vi "ARCHIVE ITEM.vi"(10 "REFERENCES":T2, 11 "ITEM DATA IN":T1) -> ()   [LabVIEW 2019]
uses:
  Controls/References Cluster.ctl
  <vilib>/userDefined/High Color/IMAQdx.ctl
  Controls/Custom Calendar/Custom Calendar.xctl
  Controls/Table Data Types/Inventory Archive Data Type.ctl
  Controls/Table Data Types/Checked In Archive Data Type.ctl
  <vilib>/addons/database/Connection.llb/DB Tools Open Connec (String).vi
  <vilib>/addons/database/NI_Database_API.lvlib
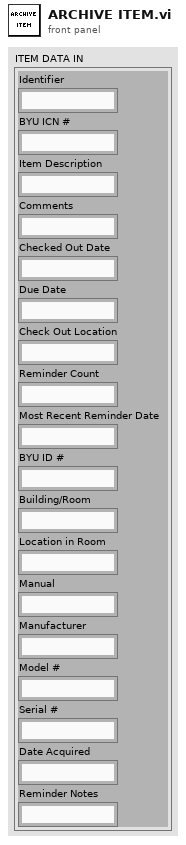
[diagram p1: front panel]
types:
  T1 = cluster{"Identifier":string, "BYU ICN #":string, "Item Description":string, "Comments":string, "Checked Out Date":string, "Due Date":string, "Check Out Location":string, "Reminder Count":string, "Most Recent Reminder Date":string, "BYU ID #":string, "Building/Room":string, "Location in Room":string, "Manual":string, "Manufacturer":string, "Model #":string, "Serial #":string, "Date Acquired":string, "Reminder Notes":string}
  T2 = typedef "References Cluster.ctl" = cluster{"MAIN PAGES":refnum<vi>, "ADD/EDIT ITEM REFERENCES":cluster{"Identifier":refnum<vi>, "BYU ICN #":refnum<vi>, "Item Description":refnum<vi>, "Comments":refnum<vi>, "Checked Out Date":refnum<vi>, "Due Date":refnum<vi>, "Check Out Location":refnum<vi>, "Reminder Count":refnum<vi>, "Most Recent Reminder Date":refnum<vi>, "BYU ID #":refnum<vi>, "Building/Room":refnum<vi>, "Location in Room":refnum<vi>, "Manual":refnum<vi>, "Manufacturer":refnum<vi>, "Model #":refnum<vi>, "Serial #":refnum<vi>, "Date Acquired":refnum<vi>, "ADD/EDIT ITEM LABEL":refnum<vi>, "ARCHIVE ITEM":refnum<vi>, "Archive Item Inputs":refnum<vi>, "Reminder Notes":refnum<vi>}, "ADD/EDIT USER REFERENCES":cluster{"BYU ID # (##-###-####)":refnum<vi>, "First Name":refnum<vi>, "Last Name":refnum<vi>, "Phone Number (###-###-####)":refnum<vi>, "Email":refnum<vi>, "Department":refnum<vi>, "Graduation Status":refnum<vi>, "Anticipated Graduation Year":refnum<vi>, "Credit Score":refnum<vi>, "Date Added":refnum<vi>, "Graduation Clearance Date":refnum<vi>, "Picture File Name":refnum<vi>, "ADD/EDIT USER LABEL":refnum<vi>, "Department Map":refnum<vi>, "Status Map":refnum<vi>, "Anticipated Graduation Year Map":refnum<vi>, "User Agreement":refnum<vi>, "User Comments":refnum<vi>, "Camera":refnum<vi>}, "RETURN ITEM REFERENCES":cluster{"Item or Person:":refnum<vi>, "Search Return Results":refnum<vi>, "What are you searching for?":refnum<vi>}, "SEARCH DATABASE REFERENCES":cluster{"What to Search For:":refnum<vi>, "Where to Search":refnum<vi>, "Column to Search In":refnum<vi>, "Column to Sort By":refnum<vi>, "Search Database Results":refnum<vi>, "Inventory Column Selector":refnum<vi>, "User Column Selector":refnum<vi>, "Inventory Archive Column Selector":refnum<vi>, "User Archive Column Selector":refnum<vi>, "Sales Tracking Column Selector":refnum<vi>, "Checked In Archive Column Selector":refnum<vi>, "Restore User":refnum<vi>, "Date Range":refnum<vi>, "Dates Less Than":refnum<vi>, "Dates Greater Than":refnum<vi>, "Search Print Receipt":refnum<vi>, "Edit Sale Description":refnum<vi>}, "USER ITEMS REFERENCES":cluster{"USER'S INFORMATION":refnum<vi>, "User's Checked Out Items":refnum<vi>, "User Info Comments":refnum<vi>, "SEE USER INFO COMMENTS":refnum<vi>}, "EDIT ITEMS REFERENCES":cluster{"New Check Out Location":refnum<vi>, "Items to Edit":refnum<vi>, "Edit Items Due Date":refnum<vi>, "New Reminder Notes":refnum<vi>, "New Item Description":refnum<vi>}, "CHECK OUT ITEMS REFERENCES":cluster{"Enter Item:":refnum<vi>, "Check Out Items Due Date":refnum<vi>, "Check Out Location":refnum<vi>, "Items to be Checked Out":refnum<vi>, "Possible Items":refnum<vi>, "Altered Item Description":refnum<vi>}, "TRANSFER ITEMS REFERENCES":cluster{"Search Parameter":refnum<vi>, "What to Match":refnum<vi>, "Matching Individuals":refnum<vi>, "Items to be Transferred":refnum<vi>}, "SETTINGS REFERENCES":cluster{"PSC Database Settings":refnum<vi>, "PSC Sales Item Spreadsheet":refnum<vi>}, "PSC SALES REFERENCES":cluster{"BYU ID CARD #":refnum<vi>, "Sale Description":refnum<vi>, "Scan or Enter Item Name":refnum<vi>, "Items to be Sold":refnum<vi>, "Grand Total":refnum<vi>, "Item List":refnum<vi>}}
  T3 = typedef "Inventory Archive Data Type.ctl" = cluster{"Date Disposed":string, "Disposal Method":string, "Auction #":string, "Date Inventory Office Emailed":string, "Disposal Notes":string, "Identifier":string, "BYU ICN #":string, "Item Description":string, "Comments":string, "Building/Room":string, "Location in Room":string, "Manual":string, "Manufacturer":string, "Model #":string, "Serial #":string, "Date Acquired":string}
  T4 = cluster{"Identifier":refnum<vi>, "BYU ICN #":refnum<vi>, "Item Description":refnum<vi>, "Comments":refnum<vi>, "Checked Out Date":refnum<vi>, "Due Date":refnum<vi>, "Check Out Location":refnum<vi>, "Reminder Count":refnum<vi>, "Most Recent Reminder Date":refnum<vi>, "BYU ID #":refnum<vi>, "Building/Room":refnum<vi>, "Location in Room":refnum<vi>, "Manual":refnum<vi>, "Manufacturer":refnum<vi>, "Model #":refnum<vi>, "Serial #":refnum<vi>, "Date Acquired":refnum<vi>, "ADD/EDIT ITEM LABEL":refnum<vi>, "ARCHIVE ITEM":refnum<vi>, "Archive Item Inputs":refnum<vi>, "Reminder Notes":refnum<vi>}
  T5 = typedef "NI_Database_API.lvlib/Conn ObjectReference.ctl" = refnum<k1>
  T6 = typedef "Checked In Archive Data Type.ctl" = cluster{"Identifier":string, "BYU ICN #":string, "Item Description":string, "Comments":string, "Checked Out Date":string, "Due Date":string, "Check Out Location":string, "Reminder Count":i32, "Most Recent Reminder Date":string, "BYU ID #":string, "Building/Room":string, "Location in Room":string, "Manual":string, "Manufacturer":string, "Model #":string, "Serial #":string, "Date Acquired":string, "Date Returned":string, "Reminder Notes":string}
  T7 = cluster{"Disposal Date":string, "Disposal Method":u16, "Auction # / Other":string, "Date Disposal Email Sent":string, "Disposal Notes":string}
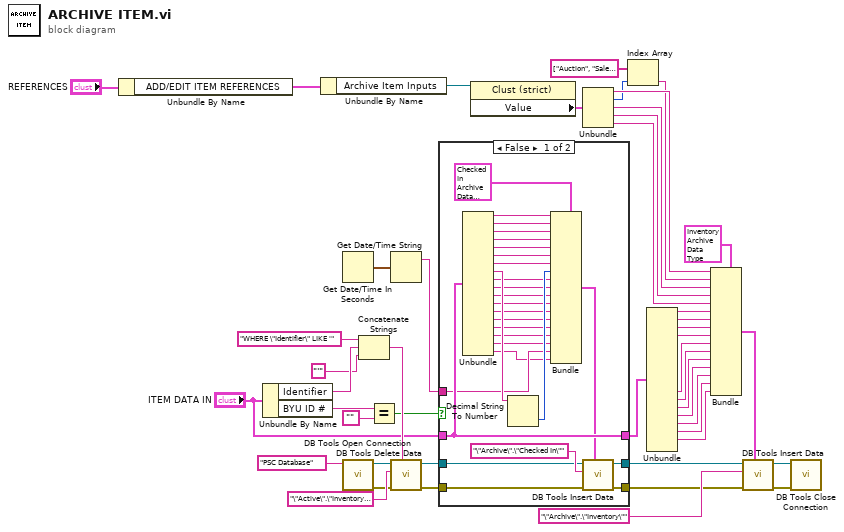
[diagram p0: block diagram]
diagram:
  n1 = Unbundle By Name("REFERENCES") -> ("ADD/EDIT ITEM REFERENCES"=w27:T4)
  n2 = Unbundle By Name("ITEM DATA IN") -> ("Identifier"=w44:string, "BYU ID #"=w39:string)
  n3 = Unbundle By Name(w27) -> ("Archive Item Inputs"=w26:refnum<vi>)
  n4 = Get Date/Time In Seconds() -> (seconds since 1Jan1904=w29:timestamp)
  n5 = call-poly <vilib>:"DB Tools Open Connection.vi"("connection information"="PSC Database") -> ("error out"=w41:errorcluster, "connection reference"=w40:T5)  [unwired: 7 in]
  n6 = Concatenate Strings("WHERE \"Identifier\" LIKE '" ("string"), w44, "'" ("string")) -> (w43:string)
  n7 = Equal?(x=w39, y="") -> (x = y?=w37:bool)
  n8 = Get Date/Time String(seconds (now)=w29) -> (date string=w28:string)  [unwired: 2 in, 1 out]
  n9 = call <vilib>:"DB Tools Delete Data.vi"("condition"=w43, "error in (no error)"=w41, "table"="\"Active\".\"Inventory\"" ("string"), "connection reference"=w40) -> ("error out"=w35:errorcluster, "connection reference out"=w36:T5)  [unwired: 6 in]
  n10 = case shown="False" w37 {
    tunnel: w36 -> [w73 w77]
    tunnel: w35 -> [w72 w76]
    tunnel: [w71 w77] -> w32
    tunnel: [w70 w76] -> w33
    tunnel: "ITEM DATA IN" -> [w69 w75]
    tunnel: [w69 w75] -> w24
    tunnel: w28 -> [w48 _]
    frame False {
      n11 = Unbundle(w69) -> ("Identifier"=w66:string, "BYU ICN #"=w65:string, "Item Description"=w64:string, "Comments"=w63:string, "Checked Out Date"=w62:string, "Due Date"=w61:string, "Check Out Location"=w60:string, "Reminder Count"=w59:string, "Most Recent Reminder Date"=w57:string, "BYU ID #"=w56:string, "Building/Room"=w55:string, "Location in Room"=w54:string, "Manual"=w53:string, "Manufacturer"=w52:string, "Model #"=w51:string, "Serial #"=w50:string, "Date Acquired"=w49:string, "Reminder Notes"=w47:string)
      n12 = Decimal String To Number(string=w59) -> (number=w58:i32)  [unwired: 2 in, 1 out]
      n13 = Bundle(cluster=T6 {"Identifier"="", "BYU ICN #"="", "Item Description"="", "Comments"="", "Checked Out Date"="", "Due Date"="", "Check Out Location"="", "Reminder Count"=0, "Most Recent Reminder Date"="", "BYU ID #"="", "Building/Room"="", "Location in Room"="", "Manual"="", "Manufacturer"="", "Model #"="", "Serial #"="", "Date Acquired"="", "Date Returned"="", "Reminder Notes"=""} ("CHECKED IN ARCHIVE DATA TYPE"), "Identifier"=w66, "BYU ICN #"=w65, "Item Description"=w64, "Comments"=w63, "Checked Out Date"=w62, "Due Date"=w61, "Check Out Location"=w60, "Reminder Count"=w58, "Most Recent Reminder Date"=w57, "BYU ID #"=w56, "Building/Room"=w55, "Location in Room"=w54, "Manual"=w53, "Manufacturer"=w52, "Model #"=w51, "Serial #"=w50, "Date Acquired"=w49, "Date Returned"=w48, "Reminder Notes"=w47) -> (w68:T6)
      n14 = call <vilib>:"DB Tools Insert Data.vi"("data"=w68, "error in (no error)"=w72, "table"="\"Archive\".\"Checked In\"" ("string"), "connection reference"=w73) -> ("error out"=w70:errorcluster, "connection reference out"=w71:T5)  [unwired: 6 in]
    }
    frame True {
    }
  }
  n15 = property class="Clust (strict)"(reference=w26) -> ("Value"=w25:T7)  [unwired: 1 in, 2 out]
  n16 = Unbundle(w25) -> ("Disposal Date"=w19:string, "Disposal Method"=w15:u16, "Auction # / Other"=w21:string, "Date Disposal Email Sent"=w22:string, "Disposal Notes"=w23:string)
  n17 = Index Array(array=string[] ["Auction", "Sale", "Surplus", "Trash", "Other"], index=w15) -> (element=w18:string)
  n18 = Unbundle(w24) -> ("Identifier"=w12:string, "BYU ICN #"=w11:string, "Item Description"=w10:string, "Comments"=w9:string, "Building/Room"=w8:string, "Location in Room"=w7:string, "Manual"=w6:string, "Manufacturer"=w5:string, "Model #"=w4:string, "Serial #"=w2:string, "Date Acquired"=w3:string)  [unwired: 7 out]
  n19 = Bundle(cluster=T3 {"Date Disposed"="", "Disposal Method"="", "Auction #"="", "Date Inventory Office Emailed"="", "Disposal Notes"="", "Identifier"="", "BYU ICN #"="", "Item Description"="", "Comments"="", "Building/Room"="", "Location in Room"="", "Manual"="", "Manufacturer"="", "Model #"="", "Serial #"="", "Date Acquired"=""} ("INVENTORY ARCHIVE DATA TYPE"), "Date Disposed"=w19, "Disposal Method"=w18, "Auction #"=w21, "Date Inventory Office Emailed"=w22, "Disposal Notes"=w23, "Identifier"=w12, "BYU ICN #"=w11, "Item Description"=w10, "Comments"=w9, "Building/Room"=w8, "Location in Room"=w7, "Manual"=w6, "Manufacturer"=w5, "Model #"=w4, "Serial #"=w2, "Date Acquired"=w3) -> (w17:T3)
  n20 = call <vilib>:"DB Tools Insert Data.vi"("data"=w17, "error in (no error)"=w33, "table"="\"Archive\".\"Inventory\"" ("string"), "connection reference"=w32) -> ("error out"=w30:errorcluster, "connection reference out"=w31:T5)  [unwired: 6 in]
  n21 = call <vilib>:"DB Tools Close Connection.vi"("error in (no error)"=w30, "connection reference"=w31) -> ()  [unwired: 5 in, 1 out]
